vi "Charger_Is Charge Error.vi"(7 "Status Refnum":T1, 8 "error in":errorcluster) -> (0 "error out":errorcluster, 4 "complete":bool)   [LabVIEW 2020]
uses:
  Charger_Status Refnum.ctl
  Drivers/Charger Test Set/Charger_Input Control.ctl
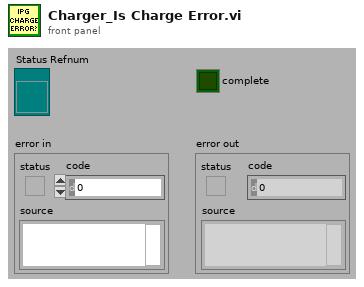
[diagram p1: front panel]
types:
  T1 = typedef "Charger_Status Refnum.ctl" = refnum<vi>
  T2 = typedef "Charger_Input Control.ctl" = cluster{"address":refnum<visa-resource-name>, "position":i32, "setpoint":dbl}
  T3 = cluster{"MICS ID":u32, "VBAT":dbl, "ChargingState":string, "VBAT Slide":dbl, "Status":string, "TemperatureLevel":dbl, "IPG_ReceivedLevel":dbl, "VBAT Target":dbl, "Charger Setpoint":dbl, "Index":i32, "Ready":bool, "Charger Inputs":T2, "MICS Inputs":cluster{"address":refnum<visa-resource-name>, "chan":u16, "ID":u32}}
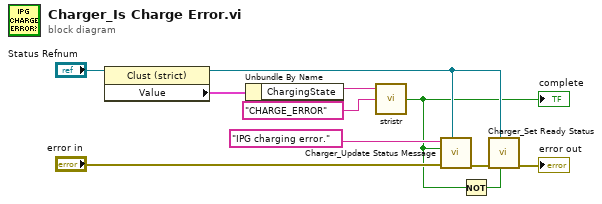
[diagram p0: block diagram]
diagram:
  n1 = property on="Status" class="Clust (strict)"(reference="Status Refnum") -> (reference out=w5:T1, "Value"=w11:T3)  [unwired: 1 in, 1 out]
  n2 = Unbundle By Name(w11) -> ("ChargingState"=w2:string)
  n3 = call "stristr.vi"("Substring"="CHARGE_ERROR" ("search string/char (-)"), "Input String"=w2) -> ("found"=w3:bool)  [unwired: 1 in, 2 out]
  "complete" <- w3
  n4 = call "Charger_Update Status Message.vi"("Status Refnum"=w5, "error in"="error in", "enable (T)"=w3, "status message"="IPG charging error." ("format string")) -> ("error out"=w9:errorcluster)  [unwired: 5 in]
  n5 = Not(x=w3) -> (.not. x?=w4:bool)
  n6 = call "Charger_Set Ready Status.vi"("Ready"=w4, "Status Refnum"=w5, "error in"=w9) -> ("error out"=→"error out":errorcluster)  [unwired: 6 in, 1 out]
